vi "Apply Panel Layout to VI.vi"(4 "defer panel updates (F)":bool, 6 "bounds (panel bounds)":T1, 7 "scaling settings":T2, 8 "error in":errorcluster, 10 "VI refnum":refnum<vi>, 11 "panel layout in":refnum<class "VI Panel Layout.lvclass">) -> (0 "error out":errorcluster, 3 "panel layout out":refnum<class "VI Panel Layout.lvclass">)   [LabVIEW 2010, in "NI_SE_Front Panel Layout.lvlib" / "VI Panel Layout.lvclass"]
doc: "Applies a panel layout to the VI. Any front panel objects in the VI will be repositioned and resized according to the panel layout description.\n\n<b>bounds</b> determines whether the panel size or the window size is used to to set the size of the VI."
uses:
  VI Panel Layout.lvclass
  Scaling Settings.ctl
  Scaling Type.ctl
  Bounds Type.ctl
  VI Panel Layout.lvclass/VI Panel Layout.ctl
  Scaling Factor_Options.ctl
  XY Scaling Factor.ctl
  Object Layout Classes/Object Layout/Object Layout.lvclass/Object Layout.ctl
  Bounds to Corner Positions.vi
  Corner Position to Bounds.vi
  Object Layout Classes/Object Layout/Get UID.vi
  Object Layout Classes/Object Layout/Get Unique Name.vi
  Convert UID To String.vi
  NI_SE_Front Panel Layout.lvlib
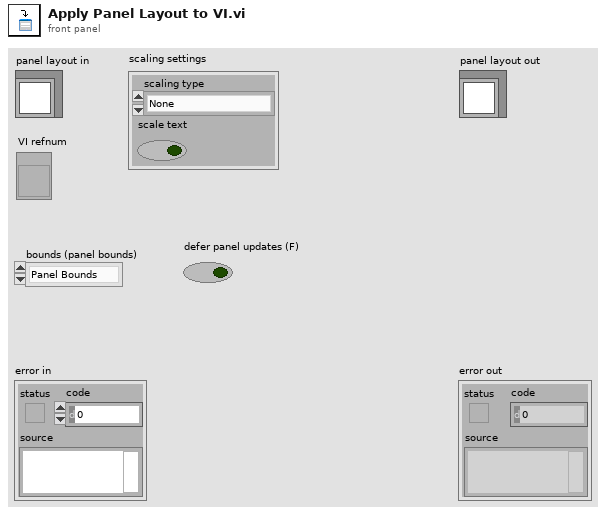
[diagram p1: front panel]
types:
  T1 = typedef "NI_SE_Front Panel Layout.lvlib/Bounds Type.ctl" = enum16{"Panel Bounds", "Window Bounds"}
  T2 = typedef "NI_SE_Front Panel Layout.lvlib/Scaling Settings.ctl" = cluster{"scaling type":T3, "scale text":bool}
  T3 = typedef "NI_SE_Front Panel Layout.lvlib/Scaling Type.ctl" = enum16{"None", "Scale panel to fit layout", "Scale layout to fit panel"}
  T4 = typedef "NI_SE_Front Panel Layout.lvlib/Scaling Factor_Options.ctl" = cluster{"scaling factor":T5, "scale text":bool}
  T5 = typedef "NI_SE_Front Panel Layout.lvlib/XY Scaling Factor.ctl" = cluster{"horizontal":dbl, "vertical":dbl}
  T6 = enum32{"Invalid", "Standard", "Closed", "Hidden", "Minimized", "Maximized"}
  T7 = typedef "LVRectTypeDef.ctl" = cluster{"Left":i16, "Top":i16, "Right":i16, "Bottom":i16}
  T8 = typedef "LVPointTypeDef.ctl" = cluster{"Horizontal":i16, "Vertical":i16}
  T9 = cluster{"Left":bool, "Top":bool, "Right":bool, "Bottom":bool}
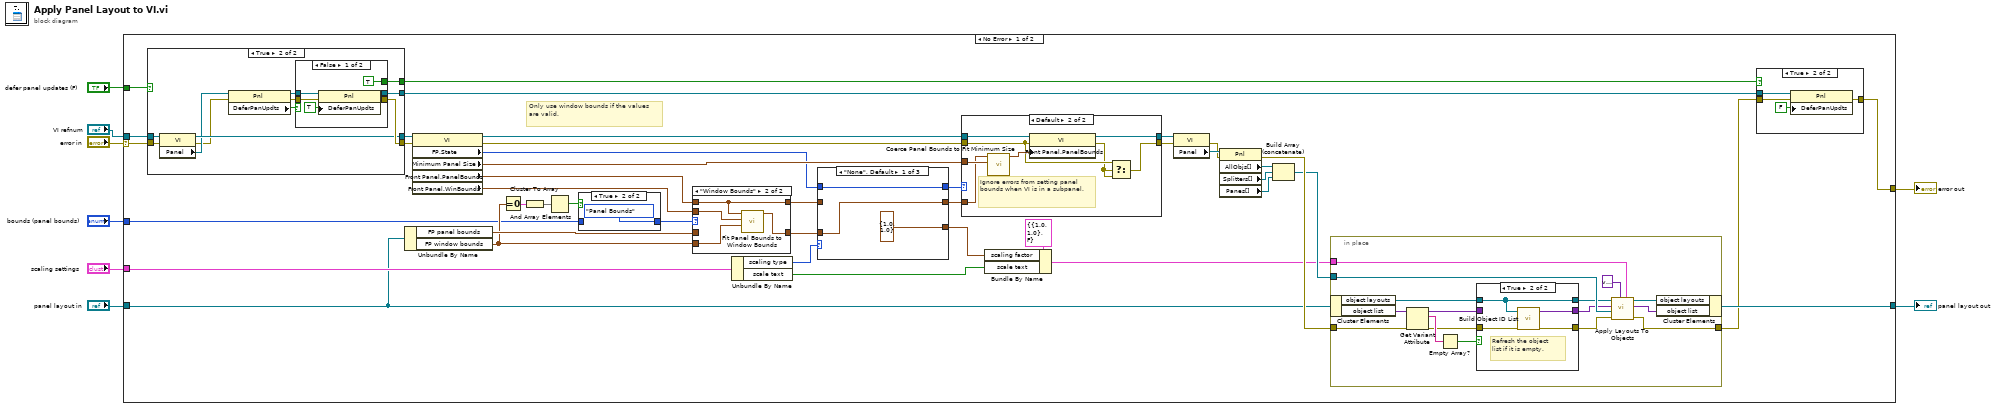
[diagram p0: block diagram]
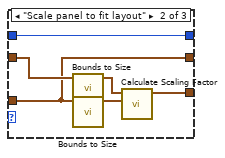
[diagram p8: hidden frame]
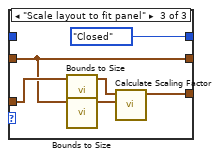
[diagram p9: hidden frame]
diagram:
  n1 = case shown="No Error" "error in" {
    selector: "error in" -> [w18 w135]
    tunnel: [w12 w135] -> w4
    tunnel: "panel layout in" -> [w21 w134]
    tunnel: [w22 w134] -> w5
    tunnel: "VI refnum" -> [w16 _]
    tunnel: "scaling settings" -> [w36 _]
    tunnel: "bounds (panel bounds)" -> [w24 _]
    tunnel: "defer panel updates (F)" -> [w11 _]
    frame No Error {
      # "Only use window bounds if the values are valid."
      n2 = case shown="True" w11 {
        tunnel: w18 -> [w57 w69]
        tunnel: [w57 w68] -> w17
        tunnel: w16 -> [w58 w67]
        tunnel: [w58 w66] -> w15
        tunnel: [_ w65] -> w14
        tunnel: [_ w59] -> w10
        frame False {
        }
        frame True {
          n3 = property class="VI"(reference=w67, error in=w69) -> (reference out=w66:refnum<vi>, error out=w62:errorcluster, "Panel"=w64:refnum<vi>)
          n4 = property class="Pnl"(reference=w64, error in=w62) -> (reference out=w63:refnum<vi>, error out=w61:errorcluster, "DeferPanUpdts"=w60:bool)
          n5 = case shown="False" w60 {
            tunnel: [w75 w76] -> w68
            tunnel: [w73 w77] -> w65
            tunnel: w63 -> [w72 w77]
            tunnel: w61 -> [w71 w76]
            tunnel: [TRUE _] -> w59
            frame False {
              n6 = property class="Pnl"(reference=w72, error in=w71, "DeferPanUpdts"=TRUE ("Defer Panel Updates")) -> (reference out=w73:refnum<vi>, error out=w75:errorcluster)
            }
            frame True {
            }
          }
        }
      }
      n7 = Unbundle By Name(w21) -> ("FP panel bounds"=w31:T7, "FP window bounds"=w28:T7)
      n8 = property class="VI"(reference=w15, error in=w17) -> (reference out=w44:refnum<vi>, error out=w43:errorcluster, "FP.State"=w20:T6, "Minimum Panel Size"=w42:T8, "Front Panel.PanelBounds"=w33:T7, "Front Panel.WinBounds"=w29:T7)
      n9 = Equal To 0?(x=w28) -> (x = 0?=w27:T9)
      n10 = Cluster To Array(cluster=w27) -> (array=w26:bool[])
      n11 = And Array Elements(Boolean array=w26) -> (logical AND=w25:bool)
      n12 = case shown="True" w25 {
        tunnel: w24 -> [w101 _]
        tunnel: [w101 Bounds_Type."Panel Bounds" ("bounds (panel bounds)")] -> w23
        frame False {
        }
        frame True {
        }
      }
      n13 = case shown="\"Window Bounds\"" w23 {
        tunnel: w33 -> [w104 w107]
        tunnel: [w104 w107] -> w32
        tunnel: w31 -> [w103 _]
        tunnel: [w103 w105] -> w30
        tunnel: w28 -> [_ w106]
        tunnel: w29 -> [_ w108]
        frame "Panel Bounds" {
        }
        frame "Window Bounds" {
          n14 = call "Fit Panel Bounds to Window Bounds.vi"("desired window bounds"=w106, "VI window bounds"=w108, "VI panel bounds"=w107) -> ("desired panel bounds"=w105:T7)  [unwired: 8 in]
        }
      }
      n15 = Unbundle By Name(w36) -> ("scaling type"=w34:T3, "scale text"=w9:bool)
      n16 = case shown="\"None\", Default" w34 {
        tunnel: w30 -> [w110 w113 w121]
        tunnel: w32 -> [_ w117 w119]
        tunnel: [T5 {"horizontal"=1.0, "vertical"=1.0} ("scaling factor") w116 w120] -> w37
        tunnel: [w110 w113 w119] -> w35
        tunnel: w20 -> [w109 w112 _]
        tunnel: [w109 w112 T6."Closed" ("FP.State")] -> w19
        frame "None", Default {
        }
        frame "Scale panel to fit layout" {
          n17 = call "Bounds to Size.vi"("bounds"=w117) -> ("size"=w114:T8)  [unwired: 10 in]
          n18 = call "Bounds to Size.vi"("bounds"=w113) -> ("size"=w115:T8)  [unwired: 10 in]
          n19 = call "Calculate Scaling Factor.vi"("desired size"=w115, "unscaled size"=w114) -> ("scaling factor"=w116:T5)  [unwired: 9 in]
        }
        frame "Scale layout to fit panel" {
          n20 = call "Bounds to Size.vi"("bounds"=w121) -> ("size"=w122:T8)  [unwired: 10 in]
          n21 = call "Bounds to Size.vi"("bounds"=w119) -> ("size"=w123:T8)  [unwired: 10 in]
          n22 = call "Calculate Scaling Factor.vi"("desired size"=w123, "unscaled size"=w122) -> ("scaling factor"=w120:T5)  [unwired: 9 in]
        }
      }
      n23 = case shown="Default" w19 {
        tunnel: [w124 w133] -> w45
        tunnel: w35 -> [_ w126]
        tunnel: [w125 w127] -> w41
        tunnel: w44 -> [w124 w132]
        tunnel: w43 -> [w125 w129]
        tunnel: w42 -> [_ w131]
        frame "Closed" {
          # "Do not set the FP bounds if the window is closed, or if scaling is set to \"Scale layout to fit panel\"."
        }
        frame Default {
          # "Ignore errors from setting panel bounds when VI is in a subpanel."
          n24 = call "Coerce Panel Bounds to Fit Minimum Size.vi"("minimum panel size"=w131, "FP panel bounds in"=w126) -> ("FP panel bounds out"=w130:T7)  [unwired: 9 in]
          n25 = property class="VI"(reference=w132, error in=w129, "Front Panel.PanelBounds"=w130) -> (reference out=w133:refnum<vi>, error out=w128:errorcluster)
          n26 = Select(t=w129, s=w128, f=w128) -> (s? t:f=w127:errorcluster)
        }
      }
      n27 = Bundle By Name(cluster=T4 {"scaling factor"={"horizontal"=1.0, "vertical"=1.0}, "scale text"=FALSE} ("scaling settings"), "scaling factor"=w37, "scale text"=w9) -> (w38:T4)
      n28 = property class="VI"(reference=w45, error in=w41) -> (error out=w50:errorcluster, "Panel"=w51:refnum<vi>)  [unwired: 1 out]
      n29 = property class="Pnl"(reference=w51, error in=w50) -> (error out=w49:errorcluster, "AllObjs[]"=w48:refnum<vi>[], "Splitters[]"=w47:refnum<vi>[], "Panes[]"=w40:refnum<vi>[])  [unwired: 1 out]
      n30 = Build Array (concatenate)(w48, w47, w40) -> (w46:refnum<vi>[])
      n31 = in-place {
        in-place-border: [w88] -> w13
        in-place-border: w49 -> [w85]
        in-place-border: w46 -> [w93]
        in-place-border: w38 -> [w92]
        n32 = in-place-cluster #1(w21) -> ("object layouts"=w81:refnum<class "Object Layout.lvclass">[], "object list"=w86:variant)
        n33 = Get Variant Attribute(Variant=w86, error in=w85) -> (duplicate Variant=w83:variant, names=w87:string[], error out=w79:errorcluster)  [unwired: 2 in, 1 out]
        n34 = Empty Array?(array=w87) -> (empty?=w84:bool)
        n35 = case shown="True" w84 {
          tunnel: w83 -> [w96 _]
          tunnel: [w96 w99] -> w82
          tunnel: w81 -> [w95 w100]
          tunnel: [w95 w100] -> w80
          tunnel: w79 -> [w94 w98]
          tunnel: [w94 w97] -> w78
          frame False {
          }
          frame True {
            # "Refresh the object list if it is empty."
            n36 = call "Build Object ID List.vi"("error in"=w98, "object layouts"=w100) -> ("error out"=w97:errorcluster, "object ID list"=w99:variant)  [unwired: 8 in]
          }
        }
        n37 = call "Apply Layouts To Objects.vi"("scaling settings"=w92, "properties to ignore"=variant, "error in"=w78, "GObj refnums"=w93, "object ID list in"=w82, "object layouts in"=w80) -> ("error out"=w88:errorcluster, "object ID list out"=w89:variant, "object layouts out"=w90:refnum<class "Object Layout.lvclass">[])  [unwired: 3 in]
        n38 = in-place-cluster #1("object layouts"=w90, "object list"=w89) -> (w22:refnum<class "VI Panel Layout.lvclass">)
      }
      n39 = case shown="True" w10 {
        tunnel: [w52 w56] -> w12
        tunnel: w14 -> [_ w54]
        tunnel: w13 -> [w52 w53]
        frame False {
        }
        frame True {
          n40 = property class="Pnl"(reference=w54, error in=w53, "DeferPanUpdts"=FALSE ("Defer Panel Updates")) -> (error out=w56:errorcluster)  [unwired: 1 out]
        }
      }
    }
    frame Error {
    }
  }
  "error out" <- w4
  "panel layout out" <- w5
